vi "Init_All_AE.vi"(7 "Flat File Path":path=path "C:/Users/STED/Desktop/Cambridge STED Control Software/Host VIs/SLM/Flatness Correction LSH0700935/CAL_LSH0700935_770nm.bmp", 8 "HoloArray In":T1[](array[typedef]), 11 "General Setting":T4 {"Mode Matrix" items=["Number", "Name"]}) -> (0 "Holo Array Out":T1[](array[typedef]))   [LabVIEW 2018]
uses:
  Controls/Holo Setting.ctl
  Controls/Buttons/Running Button.ctl
  Controls/Zernike Polynominals.ctl
  Controls/General Setting.ctl
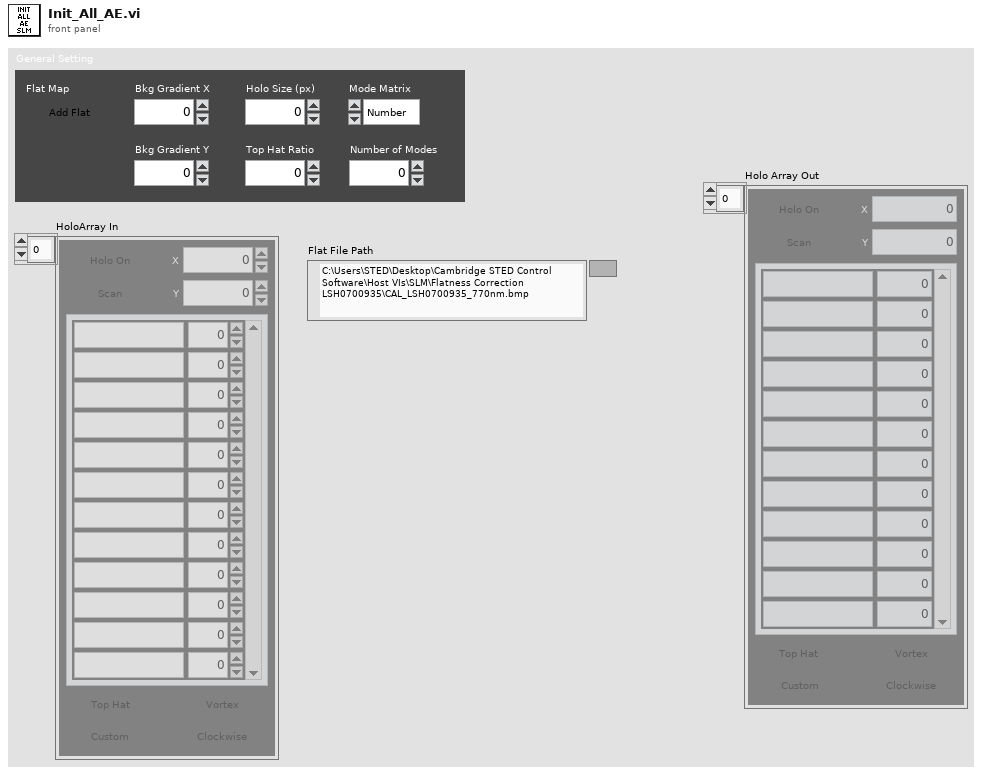
[diagram p1: front panel]
types:
  T1 = typedef "Holo Setting.ctl" = cluster{"Holo On":T2, "Scan":T2, "X":i16, "Y":i16, "Zernike Polynominals":T3, "Top Hat":T2, "Vortex":T2, "Clockwise":T2, "Custom":T2}
  T2 = typedef "Running Button.ctl" = bool
  T3 = typedef "Zernike Polynominals.ctl" = cluster{"Aberration Name":string, "Numeric":dbl}[]
  T4 = typedef "General Setting.ctl" = cluster{"Flat Map":T2, "Bkg Gradient X":dbl, "Bkg Gradient Y":dbl, "Holo Size (px)":i32, "Top Hat Ratio":dbl, "Number of Modes":i8, "Mode Matrix":u16}
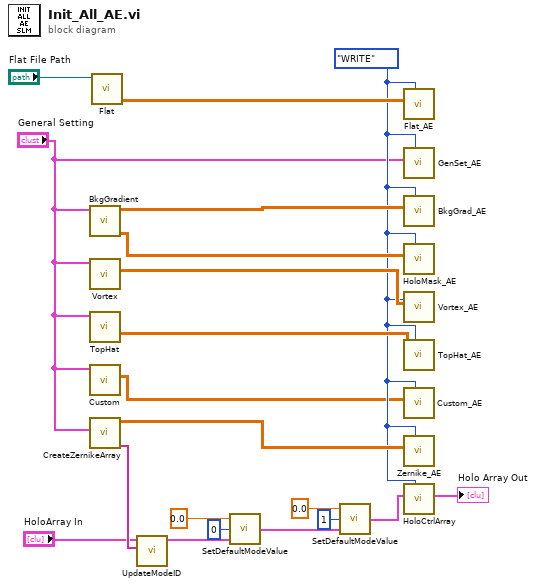
[diagram p0: block diagram]
diagram:
  w3 = enum16{"READ", "WRITE"}."WRITE" ("Action")
  n1 = call "BkgGradient.vi"("General settings"="General Setting") -> ("Holo mask"=w13:dbl[][], "gradient"=w12:dbl[][])  [unwired: 9 in]
  n2 = call "Vortex.vi"("General settings"="General Setting") -> ("Vortex"=w17:dbl[][])  [unwired: 10 in]
  n3 = call "TopHat.vi"("General settings"="General Setting") -> ("TopHat"=w16:dbl[][])  [unwired: 10 in]
  n4 = call "Custom.vi"("General settings"="General Setting") -> ("Vortex"=w2:dbl[][])  [unwired: 10 in]
  n5 = call "CreateZernikeArray.vi"("General settings"="General Setting") -> ("Mode IDs"=w14:string[], "Modes Out"=w15:dbl[][][])  [unwired: 9 in]
  n6 = call "Flat.vi"("File Path"="Flat File Path") -> ("Flatness"=w20:dbl[][])  [unwired: 10 in]
  n7 = call "UpdateModeID.vi"("Mode IDs"=w14, "Array in"="HoloArray In") -> ("Array out"=w11:T1[])  [unwired: 9 in]
  n8 = call "SetDefaultModeValue.vi"("Array in"=w11, "index"=0, "Amplititute"=0.0) -> ("output array"=w8:T1[])
  n9 = call "SetDefaultModeValue.vi"("Array in"=w8, "index"=1, "Amplititute"=0.0) -> ("output array"=w5:T1[])
  n10 = call "Flat_AE.vi"("Action"=w3, "Flat In"=w20) -> ()  [unwired: 9 in, 1 out]
  n11 = call "GenSet_AE.vi"("Enum"=w3, "General settings"="General Setting") -> ()  [unwired: 9 in, 1 out]
  n12 = call "BkgGrad_AE.vi"("Action"=w3, "BkgGrad In"=w12) -> ()  [unwired: 9 in, 1 out]
  n13 = call "HoloMask_AE.vi"("Action"=w3, "HoloMask In"=w13) -> ()  [unwired: 9 in, 1 out]
  n14 = call "Vortex_AE.vi"("Action"=w3, "Vortex In"=w17) -> ()  [unwired: 9 in, 1 out]
  n15 = call "TopHat_AE.vi"("Action"=w3, "TopHat In"=w16) -> ()  [unwired: 9 in, 1 out]
  n16 = call "Custom_AE.vi"("Action"=w3, "Custom In"=w2) -> ()  [unwired: 9 in, 1 out]
  n17 = call "Zernike_AE.vi"("Action"=w3, "Zernike In"=w15) -> ()  [unwired: 9 in, 1 out]
  n18 = call "HoloCtrlArray.vi"("Action"=w3, "Holo Array In"=w5) -> ("Holo Array Out"=→"Holo Array Out":T1[])  [unwired: 9 in]
